vi "Drive Teleop.vi"(7 "New Stuff":bool, 11 "Cluster":T1) -> ()   [LabVIEW 2018]
uses:
  Support Code/Joystick Vals.ctl
  Support Code/Path Data.ctl
  Implementation/Drive Operations.ctl
  Climb/Implementation/Climb Operations.ctl
  <vilib>/Rock Robotics/Network Tables/NT Read Number.vi
  Framework/Robot Global Data.vi
  <vilib>/Rock Robotics/Network Tables/NT Read String.vi
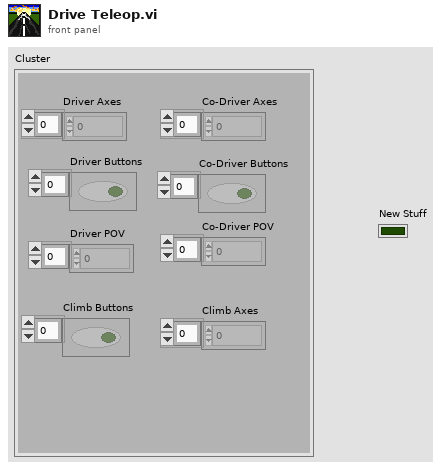
[diagram p1: front panel]
types:
  T1 = typedef "Joystick Vals.ctl" = cluster{"Driver Axes":dbl[], "Co-Driver Axes":dbl[], "Driver Buttons":bool[], "Co-Driver Buttons":bool[], "Driver POV":i16[], "Co-Driver POV":i16[], "Climb Buttons":bool[], "Climb Axes":dbl[]}
  T2 = typedef "Path Data.ctl" = cluster{"Maneuver":enum16{"MAX 90", "MAX 180", "Turn to Home", "Turn to Rocket", "Auto-Align", "Turn to ..."}, "Rotation Direction":enum16{"N/A", "Right", "Left"}}[]
  T3 = typedef "Drive Operations.ctl" = enum16{"Reserve", "Read Current", "Immediate", "J-Turn", "Play Back From Log", "Auto-Align"}
  T4 = cluster{"Reverse (T) / Normal (F)":bool, "Power Scaling (1=Normal) ":dbl, "Deadband Value":dbl}
  T5 = typedef "Drive Setpoints.ctl" = cluster{"Operation":T3, "Left Setpoint (Power)":dbl, "Right Setpoint (Turning)":dbl, "Reverse (T) / Normal (F)":bool, "Power Scaling (1=Normal) ":dbl, "Path Data":T2, "Path":path, "Angle boi":dbl, "Path Reversed":bool, "Align for Path":bool, "80A(T)/45(F)":bool, "Auto Path Data":cluster{"V":dbl[], "Theta":dbl[], "Commands":cluster{"Time into Path":dbl, "System":T6, "Item Selected?":bool, "System Selection":T6}[], "Sample Period":dbl}}
  T6 = typedef "Availible Command systems for auto.ctl" = u16
  T7 = typedef "Climb Operations.ctl" = enum16{"Reserve", "Read Current", "Immediate", "Ready", "Auto-Climb", "Reset/Turbo-Tilt", "Manual Climb"}
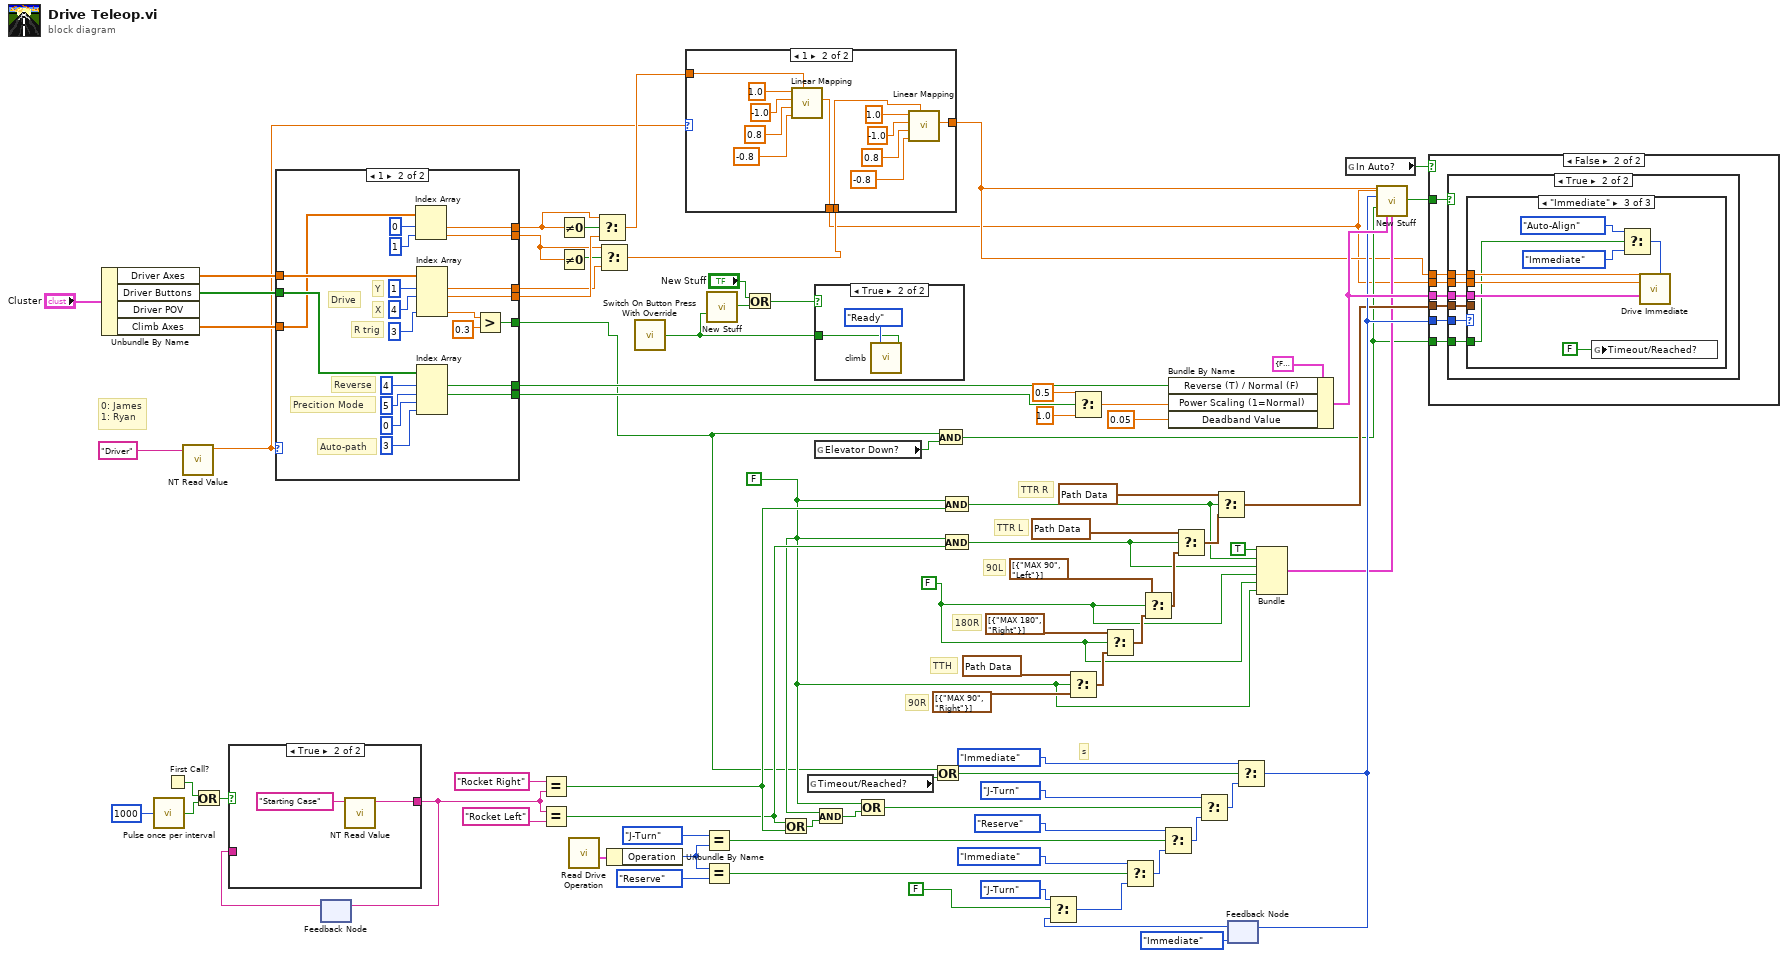
[diagram p0: block diagram]
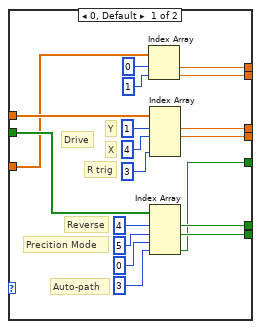
[diagram p3: hidden frame]
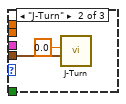
[diagram p8: hidden frame]
diagram:
  w9 = FALSE
  w15 = FALSE ("s")
  # "0: James\n1: Ryan"
  # "s"
  # "TTR L"
  # "TTR R"
  # "TTH"
  # "90R"
  # "90L"
  # "180R"
  n1 = Unbundle By Name("Cluster") -> ("Driver Axes"=w82:dbl[], "Driver Buttons"=w83:bool[], "Climb Axes"=w27:dbl[])  [unwired: 1 out]
  n2 = call "Pulse once per interval.vi"("Time (ms)"=u32 1000) -> ("Boolean"=w40:bool)
  n3 = First Call?() -> (First Call?: T/F=w42:bool)
  n4 = call-poly <vilib>:"NT Read Value.vi"("Name"="Driver") -> ("Numeric"=w3:dbl)  [unwired: 9 in, 1 out]
  n5 = Or(x=w42, y=w40) -> (x .or. y?=w41:bool)
  n6 = case shown="1" w3 {
    tunnel: w83 -> [w103 w124]
    tunnel: w82 -> [w102 w123]
    tunnel: [w97 w118] -> w78
    tunnel: [w96 w117] -> w73
    tunnel: w27 -> [w94 w115]
    tunnel: [w91 w112] -> w25
    tunnel: [w90 w111] -> w24
    tunnel: [w89 w110] -> w22
    tunnel: [w88 w109] -> w21
    tunnel: [w85 w104] -> w1
    frame 0, Default {
      # "Auto-path"
      # "R trig"
      # "Y"
      # "X"
      # "Drive"
      # "Precition Mode"
      # "Reverse"
      n7 = Index Array(array=w94, index #1=0, index #2=1) -> (element #1=w90:dbl, element #2=w89:dbl)
      n8 = Index Array(array=w102, index #1=1 ("index"), index #2=4 ("index"), index #4=3 ("index")) -> (element #1=w88:dbl, element #2=w91:dbl)  [unwired: 1 in, 2 out]
      n9 = Index Array(array=w103, index #1=4 ("index"), index #2=5 ("index"), index #3=0 ("index"), index #4=3 ("index")) -> (element #1=w97:bool, element #2=w96:bool, element #4=w85:bool)  [unwired: 1 out]
    }
    frame 1 {
      # "Auto-path"
      # "R trig"
      # "Y"
      # "X"
      # "Drive"
      # "Precition Mode"
      # "Reverse"
      n10 = Index Array(array=w115, index #1=0, index #2=1) -> (element #1=w111:dbl, element #2=w110:dbl)
      n11 = Index Array(array=w123, index #1=1 ("index"), index #2=4 ("index"), index #4=3 ("index")) -> (element #1=w109:dbl, element #2=w112:dbl, element #4=w105:dbl)  [unwired: 1 in, 1 out]
      n12 = Index Array(array=w124, index #1=4 ("index"), index #2=5 ("index"), index #3=0 ("index"), index #4=3 ("index")) -> (element #1=w118:bool, element #2=w117:bool)  [unwired: 2 out]
      n13 = Greater?(x=w105, y=0.3) -> (0:w104:bool)
    }
  }
  n14 = feedback #1() -> (w43:string)  [unwired: 1 in]
  n15 = case shown="True" w41 {
    tunnel: [w125 w127] -> w44
    tunnel: w43 -> [w125 _]
    frame False {
    }
    frame True {
      n16 = call-poly <vilib>:"NT Read Value.vi"("Name"="Starting Case") -> ("String"=w127:string)  [unwired: 9 in, 1 out]
    }
  }
  n17 = feedback-in #1(w44) -> ()
  n18 = Equal?(x="Rocket Right", y=w44) -> (x = y?=w47:bool)
  n19 = Equal?(x=w44, y="Rocket Left") -> (x = y?=w46:bool)
  n20 = Not Equal To 0?(x=w24) -> (x != 0?=w26:bool)
  n21 = Not Equal To 0?(x=w22) -> (x != 0?=w23:bool)
  n22 = call "Read Drive Operation.vi"() -> ("SubSystem Data"=w72:T5)  [unwired: 9 in, 2 out]
  n23 = Select(t=w24, s=w26, f=w25) -> (s? t:f=w5:dbl)
  n24 = Select(t=w22, s=w23, f=w21) -> (s? t:f=w7:dbl)
  n25 = Unbundle By Name(w72) -> ("Operation"=w38:T3)
  n26 = call "Switch On Button Press With Override.vi"() -> ("Output"=w14:bool)  [unwired: 3 in]
  n27 = case shown="1" w3 {
    tunnel: w7 -> [w128 w133]
    tunnel: [w128 w132] -> w6
    tunnel: w5 -> [w129 w131]
    tunnel: [w129 w130] -> w4
    frame 0, Default {
    }
    frame 1 {
      n28 = call "Linear Mapping.vi"("X"=w131, "Min B"=-0.8, "Max B"=0.8, "Min A"=-1.0, "Max A"=1.0) -> ("Y"=w130:dbl)  [unwired: 6 in]
      n29 = call "Linear Mapping.vi"("X"=w133, "Min B"=-0.8, "Max B"=0.8, "Min A"=-1.0, "Max A"=1.0) -> ("Y"=w132:dbl)  [unwired: 6 in]
    }
  }
  n30 = Equal?(x=Drive_Operations."J-Turn" ("Operation"), y=w38) -> (x = y?=w69:bool)
  n31 = Equal?(x=w38, y=Drive_Operations."Reserve" ("Operation")) -> (x = y?=w59:bool)
  n32 = call "New Stuff.vi"("Variant 15"=w14) -> ("x != y?"=w13:bool)  [unwired: 26 in]
  n33 = Or(x="New Stuff", y=w13) -> (x .or. y?=w11:bool)
  n34 = Or(x=w46, y=w47) -> (x .or. y?=w45:bool)
  n35 = global read "Robot Global Data.vi" "Timeout/Reached?"() -> (w29:bool)
  n36 = case shown="True" w11 {
    tunnel: w14 -> [_ w142]
    frame False {
    }
    frame True {
      n37 = call "climb.vi"("Operation"=Climb_Operations."Ready", "Defense mode?"=w142) -> ()  [unwired: 13 in, 1 out]
    }
  }
  n38 = global read "Robot Global Data.vi" "Elevator Down?"() -> (w17:bool)
  n39 = And(x=w15, y=w45) -> (x .and. y?=w37:bool)
  n40 = Compound Arithmetic op=OR(w15, w37) -> (w31:bool)
  n41 = Or(x=w1, y=w29) -> (x .or. y?=w30:bool)
  n42 = And(x=w1, y=w17) -> (x .and. y?=w16:bool)
  n43 = And(x=w15, y=w47) -> (x .and. y?=w35:bool)
  n44 = And(x=w15, y=w46) -> (x .and. y?=w34:bool)
  n45 = Select(t=T2 [{"Maneuver"=enum."Turn to Home", "Rotation Direction"=enum."Right"}] ("J Turn Data"), s=w15, f=T2 [{"Maneuver"=enum."MAX 90", "Rotation Direction"=enum."Right"}] ("J Turn Data")) -> (s? t:f=w63:T2)
  n46 = Select(t=0.5, s=w73, f=1.0) -> (s? t:f=w77:dbl)
  n47 = Select(t=T2 [{"Maneuver"=enum."MAX 180", "Rotation Direction"=enum."Right"}] ("J Turn Data"), s=w9, f=w63) -> (s? t:f=w76:T2)
  n48 = Select(t=T2 [{"Maneuver"=enum."MAX 90", "Rotation Direction"=enum."Left"}] ("J Turn Data"), s=w9, f=w76) -> (s? t:f=w51:T2)
  n49 = Bundle By Name(cluster=T4 {"Reverse (T) / Normal (F)"=FALSE, "Power Scaling (1=Normal) "=0.0, "Deadband Value"=0.01} ("Modifiers"), "Reverse (T) / Normal (F)"=w78, "Power Scaling (1=Normal)"=w77, "Deadband Value"=0.05) -> (w33:T4)
  n50 = Select(t=T2 [{"Maneuver"=enum."Turn to Rocket", "Rotation Direction"=enum."Left"}] ("J Turn Data"), s=w34, f=w51) -> (s? t:f=w50:T2)
  n51 = Select(t=T2 [{"Maneuver"=enum."Turn to Rocket", "Rotation Direction"=enum."Right"}] ("J Turn Data"), s=w35, f=w50) -> (s? t:f=w20:T2)
  n52 = feedback #2(Drive_Operations."Immediate" ("Operation")) -> (w65:T3)
  n53 = Select(t=Drive_Operations."J-Turn" ("Operation"), s=FALSE, f=w65) -> (s? t:f=w10:T3)
  n54 = Select(t=Drive_Operations."Immediate" ("Operation"), s=w59, f=w10) -> (s? t:f=w57:T3)
  n55 = Select(t=Drive_Operations."Reserve" ("Operation"), s=w69, f=w57) -> (s? t:f=w68:T3)
  n56 = Select(t=Drive_Operations."J-Turn" ("Operation"), s=w31, f=w68) -> (s? t:f=w53:T3)
  n57 = Select(t=Drive_Operations."Immediate", s=w30, f=w53) -> (s? t:f=w32:T3)
  n58 = feedback-in #2(w32) -> ()
  n59 = Bundle(TRUE, w35, w34, w9, w9, "s"=w15) -> (w18:cluster{bool, bool, bool, bool, bool, "s":bool})  [unwired: 1 in]
  n60 = global read "Robot Global Data.vi" "In Auto?"() -> (w28:bool)
  n61 = call "New Stuff.vi"("Variant"=w6, "Variant 2"=w4, "Variant 4"=w32, "Variant 15"=w16, "Variant 13"=w33, "Variant 6"=w18) -> ("x != y?"=w36:bool)  [unwired: 21 in]
  n62 = case shown="False" w28 {
    tunnel: w20 -> [_ w150]
    tunnel: w36 -> [_ w149]
    tunnel: w6 -> [_ w148]
    tunnel: w4 -> [_ w147]
    tunnel: w33 -> [_ w146]
    tunnel: w32 -> [_ w145]
    tunnel: w16 -> [_ w144]
    frame True {
    }
    frame False {
      n63 = case shown="True" w149 {
        tunnel: w146 -> [_ w156]
        tunnel: w147 -> [_ w155]
        tunnel: w148 -> [_ w154]
        tunnel: w145 -> [_ w153]
        tunnel: w150 -> [_ w152]
        tunnel: w144 -> [_ w151]
        frame False {
        }
        frame True {
          n64 = case shown="\"Immediate\"" w153 {
            tunnel: w156 -> [_ _ w164]
            tunnel: w154 -> [_ _ w165]
            tunnel: w155 -> [_ _ w166]
            tunnel: w152 -> [_ w158 _]
            tunnel: w151 -> [_ _ w162]
            frame "Reserve", Default {
            }
            frame "J-Turn" {
              n65 = call "J-Turn.vi"("Path Data"=w158, "Angle boi"=0.0) -> ()  [unwired: 9 in, 1 out]
            }
            frame "Immediate" {
              n66 = global write "Robot Global Data.vi" "Timeout/Reached?"(FALSE ("Timeout")) -> ()
              n67 = Select(t=Drive_Operations."Auto-Align" ("Operation"), s=w162, f=Drive_Operations."Immediate" ("Operation")) -> (s? t:f=w159:T3)
              n68 = call "Drive Immediate.vi"("Operation"=w159, "Modifiers"=w164, "Right Setpoint (Turning)"=w166, "Left Setpoint (Power)"=w165) -> ()  [unwired: 7 in, 1 out]
            }
          }
        }
      }
    }
  }
